vi "Vision Process.vi"(6 "Match Geometric Pattern 2 Setup Data":string, 7 "Tote Color":T4={"Hue"={23.67058792990901, 48.923317529462665}, "Sat"={66.78571428571429, 255.0}, "Val"={48.571428571428584, 255.0}} {"Hue" scale=0.0..255.0 scale format="%#_3g"}, 8 "Gray":T2, 9 "Template":T2, 10 "Mask":T2, 11 "Camera In":T2) -> (1 "Particles":i32, 2 "Found Totes":T1(array[cluster]) {"Normalized Rect"."Numeric 5" format="%#_2g"; "Normalized Rect"."Numeric 3" format="%#_2g"; "Normalized Rect"."Numeric 2" format="%#_2g"; "Normalized Rect"."Numeric" format="%#_2g"}, 3 "Sorted Scores":T3(array[cluster]) {"Correlation" format="%#_3g"; "Scale %" format="%#_3g"; "Score" format="%#_3g"})   [LabVIEW 2014]
uses:
  <vilib>/vision/Image Controls.llb/IMAQ Image.ctl
  Program Files (x86)/National Instruments/LabVIEW 2014/examples/FRC/roboRIO/Vision/2015 Vision Example/Vision Support Code/Camera Types.ctl
  <vilib>/vision/NI_Vision_Development_Module.lvlib
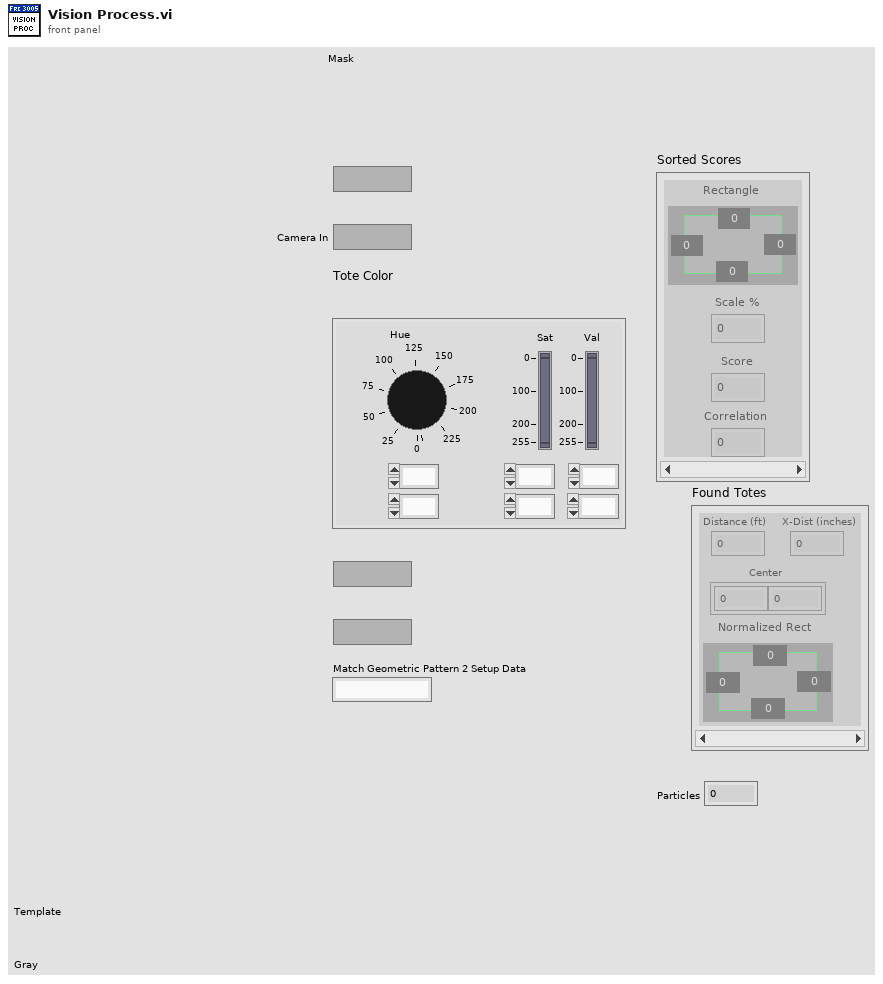
[diagram p1: front panel]
types:
  T1 = cluster{"Distance (ft)":dbl, "X-Dist (inches)":dbl, "Center":cluster{dbl, dbl}, "Normalized Rect":cluster{"Numeric":dbl, "Numeric 2":dbl, "Numeric 3":dbl, "Numeric 5":dbl}}[]
  T2 = typedef "IMAQ Image.ctl" = refnum<image>
  T3 = cluster{"Rectangle":cluster{"Numeric":dbl, "Numeric 2":dbl, "Numeric 3":dbl, "Numeric 5":dbl}, "Scale %":dbl, "Score":dbl, "Correlation":dbl}[]
  T4 = cluster{"Hue":cluster{dbl, dbl}, "Sat":cluster{dbl, dbl}, "Val":cluster{dbl, dbl}}
  T5 = typedef "Camera Types.ctl" = enum16{"206", "1011", "1013", "MS HD3000 square", "MS HD3000 640x480"}
  T6 = typedef "Particle Parameters" = i32
  T7 = cluster{"[0]":dbl, "[1]":dbl, "[2]":dbl, "[3]":dbl}
  T8 = cluster{"[0]":dbl, "[1]":dbl, "[2]":dbl, "[3]":dbl, "[4]":dbl}
  T9 = typedef "ROI Descriptor" = cluster{"Global Rectangle":i32[], "Contours":cluster{"ID":enum32{"External", "Internal"}, "Type":u32, "Coordinates":i32[]}[]}
  T10 = typedef "IMAQ GM Match Report.ctl" = cluster{"Position":cluster{"x":sgl, "y":sgl}, "Angle":sgl, "Scale":sgl, "Score":sgl, "Bounding Box":cluster{"x":sgl, "y":sgl}[], "Contrast Reversed":bool, "Occlusion %":sgl, "Template Target Curve Score":sgl, "Target Template Curve Score":sgl, "Correlation Score":sgl}
  T11 = cluster{cluster{"[0]":dbl, "[1]":dbl, "[2]":dbl, "[3]":dbl}, "Position":cluster{"x":sgl, "y":sgl}, "Bounding Box":cluster{"x":sgl, "y":sgl}[], "Scale":sgl, "Score":sgl, "Correlation Score":sgl}
  T12 = cluster{"Rectangle":cluster{"Numeric":dbl, "Numeric 2":dbl, "Numeric 3":dbl, "Numeric 5":dbl}, "Scale":dbl, "Score":dbl, "Correlation":dbl}[]
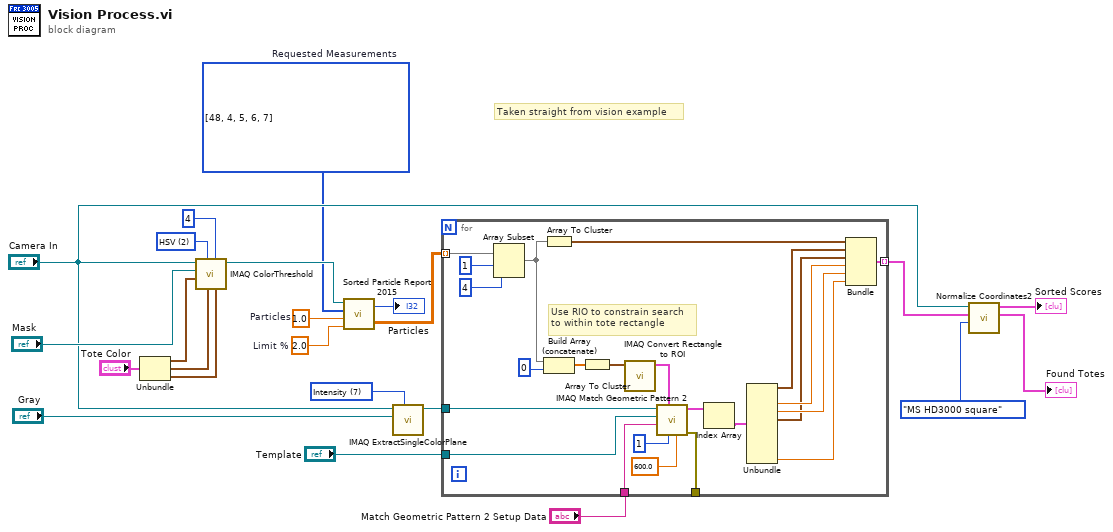
[diagram p0: block diagram]
diagram:
  w2 = T6[] [48, 4, 5, 6, 7] items=["Center of Mass X", "Center of Mass Y", "First Pixel X", "First Pixel Y", "Bounding Rect Left", "Bounding Rect Top", "Bounding Rect Right", "Bounding Rect Bottom", "Max Feret Diameter Start X", "Max Feret Diameter Start Y", "Max Feret Diameter End X", "Max Feret Diameter End Y", "Max Horiz. Segment Length Left", "Max Horiz. Segment Length Right", "Max Horiz. Segment Length Row", "-", "Bounding Rect Width", "Bounding Rect Height", "Bounding Rect Diagonal", "Perimeter", "Convex Hull Perimeter", "Holes' Perimeter", "Max Feret Diameter", "Equivalent Ellipse Major Axis", "Equivalent Ellipse Minor Axis", "Equivalent Ellipse Minor Axis (Feret)", "Equivalent Rect Long Side", "Equivalent Rect Short Side", "Equivalent Rect Diagonal", "Equivalent Rect Short Side (Feret)", "Average Horiz. Segment Length", "Average Vert. Segment Length", "Hydraulic Radius", "Waddel Disk Diameter", "-", "Area", "Holes' Area", "Particle & Holes' Area", "Convex Hull Area", "Image Area", "-", "Number of Holes", "Number of Horiz. Segments", "Number of Vert. Segments", "-", "Orientation", "Max Feret Diameter Orientation", "-", "% Area/Image Area", "% Area/(Particle & Holes' Area)", "Ratio of Equivalent Ellipse Axes", "Ratio of Equivalent Rect Sides", "-", "Elongation Factor", "Compactness Factor", "Heywood Circularity Factor", "Type Factor", "-", "Sum X", "Sum Y", "Sum XX", "Sum XY", "Sum YY", "Sum XXX", "Sum XXY", "Sum XYY", "Sum YYY", "-", "Moment of Inertia XX", "Moment of Inertia XY", "Moment of Inertia YY", "Moment of Inertia XXX", "Moment of Inertia XXY", "Moment of Inertia XYY", "Moment of Inertia YYY", "Norm. Moment of Inertia XX", "Norm. Moment of Inertia XY", "Norm. Moment of Inertia YY", "Norm. Moment of Inertia XXX", "Norm. Moment of Inertia XXY", "Norm. Moment of Inertia XYY", "Norm. Moment of Inertia YYY", "Hu Moment 1", "Hu Moment 2", "Hu Moment 3", "Hu Moment 4", "Hu Moment 5", "Hu Moment 6", "Hu Moment 7"]  # Requested Measurements
  w9 = 7 items=["Red", "Green", "Blue", "Hue", "Saturation", "Luminance", "Value", "Intensity"] ("Color Plane")
  w11 = 2.0  # Limit %
  w13 = 1.0  # Particles
  w18 = u16 2 items=["RGB", "HSL", "HSV", "HSI"] ("Color Mode")
  # "Taken straight from vision example"
  n1 = Unbundle("Tote Color") -> ("Hue"=w17:cluster{dbl, dbl}, "Sat"=w16:cluster{dbl, dbl}, "Val"=w15:cluster{dbl, dbl})
  n2 = call "IMAQ ColorThreshold"("Blue or Luma or Val or Inten Range"=w15, "Replace Value"=4, "Green or Sat Range"=w16, "Color Mode"=w18, "Red or Hue Range"=w17, "Image Dst"="Mask", "Image Src"="Camera In") -> ("Image Dst Out"=w8:T2)  [unwired: 3 in, 1 out]
  n3 = call "Sorted Particle Report 2015.vi"("Min Area Size %"=w11, "Particle Count Limit"=w13, "Pixel Measurements"=w2, "Image in"=w8) -> ("Sorted Data"=w6:dbl[][], "Particles"=→"Particles":i32)
  n4 = call "IMAQ ExtractSingleColorPlane"("Color Plane"=w9, "Image Dst"="Gray", "Image Src"="Camera In") -> ("Image Dst Out"=w7:T2)  [unwired: 7 in, 1 out]
  n5 = for {
    tunnel: w6 -> [w44] mode=indexing
    tunnel: [w43] -> w5 mode=indexing
    tunnel: w7 -> [w34]
    tunnel: "Match Geometric Pattern 2 Setup Data" -> [w36]
    tunnel: "Template" -> [w26]
    tunnel: [w25] -> _
    # "Use RIO to constrain search\nto within tote rectangle"
    n6 = Array Subset(array=w44, index=1, length=4) -> (w37:dbl[])
    n7 = Array To Cluster(array=w37) -> (cluster=w38:T7)
    n8 = Build Array (concatenate)(w37, 0 ("length")) -> (w41:dbl[])
    n9 = Array To Cluster(array=w41) -> (cluster=w40:T8)
    n10 = call "IMAQ Convert Rectangle to ROI"("Rectangle"=w40) -> ("ROI Descriptor"=w39:T9)  [unwired: 8 in, 1 out]
    n11 = call "IMAQ Match Geometric Pattern 2"("Minimum Match Score"=sgl 600.0, "Number of Matches Requested"=1 ("Minimum Match Score"), "ROI Descriptor"=w39, "Match Geometric Pattern 2 Setup Data"=w36, "Template Image"=w26, "Image"=w34) -> ("error out"=w25:errorcluster, "Matches (pixel)"=w32:T10[])  [unwired: 2 in, 2 out]
    n12 = Index Array(array=w32) -> (element=w31:T10)  [unwired: 1 in]
    n13 = Unbundle(w31) -> ("Position"=w30:cluster{"x":sgl, "y":sgl}, "Scale"=w29:sgl, "Score"=w28:sgl, "Bounding Box"=w24:cluster{"x":sgl, "y":sgl}[], "Correlation Score"=w27:sgl)  [unwired: 5 out]
    n14 = Bundle(w38, "Position"=w30, "Bounding Box"=w24, "Scale"=w29, "Score"=w28, "Correlation Score"=w27) -> (w43:T11)  [unwired: 1 in]
  }
  n15 = call "Normalize Coordinates2.vi"("Camera Type"=Camera_Types."MS HD3000 square", "Targets"=w5, "Image in"="Camera In") -> ("Found Totes"=→"Found Totes":T1, "Sorted Scores"=→"Sorted Scores":T12)  [unwired: 7 in]
